vi "Save2011.vi"   [LabVIEW 2013]
uses:
  ErrorCodes.ctl
  <vilib>/Heliosphere Research LLC/Advanced Plotting Toolkit/Advanced Plotting Toolkit.lvlib
types:
  T1 = typedef "ErrorCodes.ctl" = u32
  T2 = typedef "Advanced Plotting Toolkit.lvlib/PlotID.ctl" = i32
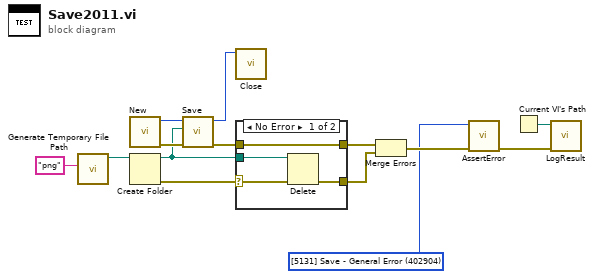
[diagram p0: block diagram]
diagram:
  w1 = T1 402904 items=["[5120] Invalid ID"=402902, "[5110] Failed to Init"=402900, "[5111] Unknown Error"=402901, "[5130] Save - Bad File Extension"=402903, "[5131] Save - General Error"=402904, "[5140] Unsupported (Polar)"=402905, "[5141] Unsupported (Logscale)"=402906, "[5142] Coordinates Not Regular"=402907] ("Expected Error")
  n1 = call <vilib>:"Generate Temporary File Path.vi"("Temporary File Extension (tmp)"="png") -> ("Unique Temporary File Path"=w8:path)  [unwired: 9 in, 1 out]
  n2 = call <vilib>:"New.vi"() -> ("error out"=w10:errorcluster, "Plot ID"=w13:T2)  [unwired: 10 in]
  n3 = Create Folder(path (use dialog)=w8) -> (created path=w6:path, error out=w7:errorcluster)  [unwired: 2 in, 1 out]
  n4 = call <vilib>:"Save.vi"("error in (no error)"=w10, "Path"=w6, "Plot ID In"=w13) -> ("error out"=w3:errorcluster, "Plot ID Out"=w12:T2)  [unwired: 7 in]
  n5 = call <vilib>:"Close.vi"("Plot ID"=w12) -> ()  [unwired: 10 in, 1 out]
  n6 = case shown="No Error" w7 {
    selector: w7 -> [w17 w20]
    tunnel: w6 -> [w18 _]
    tunnel: [w16 w20] -> w5
    tunnel: w3 -> [w15 w19]
    tunnel: [w15 w19] -> w2
    frame No Error {
      n7 = Delete(path (use dialog)=w18, error in=w17) -> (error out=w16:errorcluster)  [unwired: 3 in, 2 out]
    }
    frame Error {
    }
  }
  n8 = Merge Errors(w2, w5) -> (w4:errorcluster)
  n9 = call "AssertError.vi"("error in (no error)"=w4, "Expected Error"=w1) -> ("error out"=w11:errorcluster)  [unwired: 9 in]
  n10 = Current VI's Path() -> (path=w14:path)
  n11 = call "LogResult.vi"("Test Result"=w11, "VI Path"=w14) -> ()  [unwired: 10 in]
